vi "Continue DB Error Dialog.vi"(3 "error in (no error)":errorcluster, 4 "dialog message":string, 5 "reference":T1, 6 "connection":refnum<k7>) -> (0 "error out":errorcluster, 1 "reference":T1, 2 "connection":refnum<k7>)   [LabVIEW 2015]
doc: "Presents a dialog box that describes a database error and then continues VI execution."
uses:
  Connection - Command reference.ctl
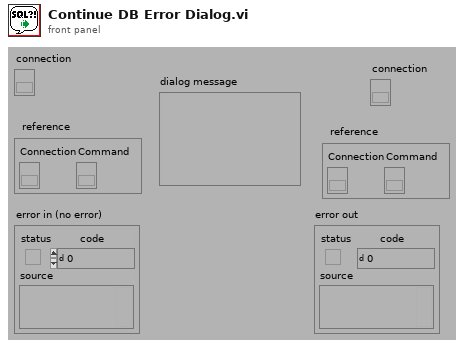
[diagram p1: front panel]
types:
  T1 = typedef "Connection - Command reference.ctl" = cluster{"Connection":refnum<k7>, "Command":refnum<k7>}
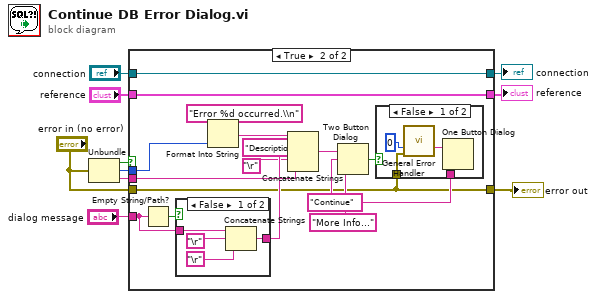
[diagram p0: block diagram]
diagram:
  n1 = Unbundle("error in (no error)") -> ("status"=w10:bool, "code"=w9:i32, "source"=w8:string)
  n2 = case shown="True" w10 {
    tunnel: w9 -> [_ w25]
    tunnel: w8 -> [_ w29]
    tunnel: [w13 w14] -> w6
    tunnel: "error in (no error)" -> [w13 w14]
    tunnel: [w11 w28] -> w5
    tunnel: "connection" -> [w11 w28]
    tunnel: [w12 w27] -> w3
    tunnel: "reference" -> [w12 w27]
    tunnel: "dialog message" -> [_ w22]
    frame False {
    }
    frame True {
      w15 = "Continue"
      n3 = Empty String/Path?(string/path=w22) -> (empty?=w23:bool)
      n4 = case shown="False" w23 {
        tunnel: w22 -> [w36 w38]
        tunnel: [w35 w38] -> w21
        frame False {
          n5 = Concatenate Strings(w36, "\r", "\r") -> (w35:string)
        }
        frame True {
        }
      }
      n6 = Format Into String(format string="Error %d occurred.\\n", w25) -> (resulting string=w24:string)  [unwired: 2 in, 1 out]
      n7 = Concatenate Strings(w24, w21, "Description:", "\r", w29) -> (w18:string)
      n8 = Two Button Dialog(message=w18, 1:"More Info...", 2:w15) -> (T button?=w16:bool)
      n9 = case shown="False" w16 {
        tunnel: w15 -> [w31 _]
        tunnel: w14 -> [w30 _]
        frame False {
          n10 = call <vilib>:"General Error Handler.vi"("type of dialog (OK msg:1)"=u16 0, "error in (no error)"=w30) -> ("message"=w32:string)  [unwired: 1 in, 12 out]
          n11 = One Button Dialog(message=w32, button name ("OK")=w31) -> ()  [unwired: 1 out]
        }
        frame True {
        }
      }
    }
  }
  "error out" <- w6
  "reference" <- w3
  "connection" <- w5
